vi "FindAccountView.vi"(1 "Exit Button":bool) -> (0 "error out":errorcluster caption="에러 출력")   [LabVIEW 2019]
uses:
  <vilib>/Utility/miscctls.llb/LVPointTypeDef.ctl
panel:
  in  "findType":enum32{"확인 버튼 2", "확인 버튼 3"}(radio)
  in  "findTab":enum32{"findIdTab", "findPwTab"}(tab)
  in  "idFindBtn":bool
  in  "idCancelBtn":bool
  in  "userNmForm":string caption="이름 *"
  in  "userEmailForm":string caption="이메일 *"
  in  "createdAtForm":string caption="가입일:"
  in  "문자열 3":string caption="아이디:"
  in  "userIdForm":string caption="아이디 *"
  in  "securityQuestion":string(combo) caption="보안 질문 선택 *"
  in  "securityAnswer":string caption="보안 질문 답변 *"
  in  "pwResetBtn":bool
  in  "pwCancelBtn":bool
  out "idChecK?":bool
  in  "정지":bool
  in  "error in (no error)":errorcluster caption="에러 입력(에러 없음)"
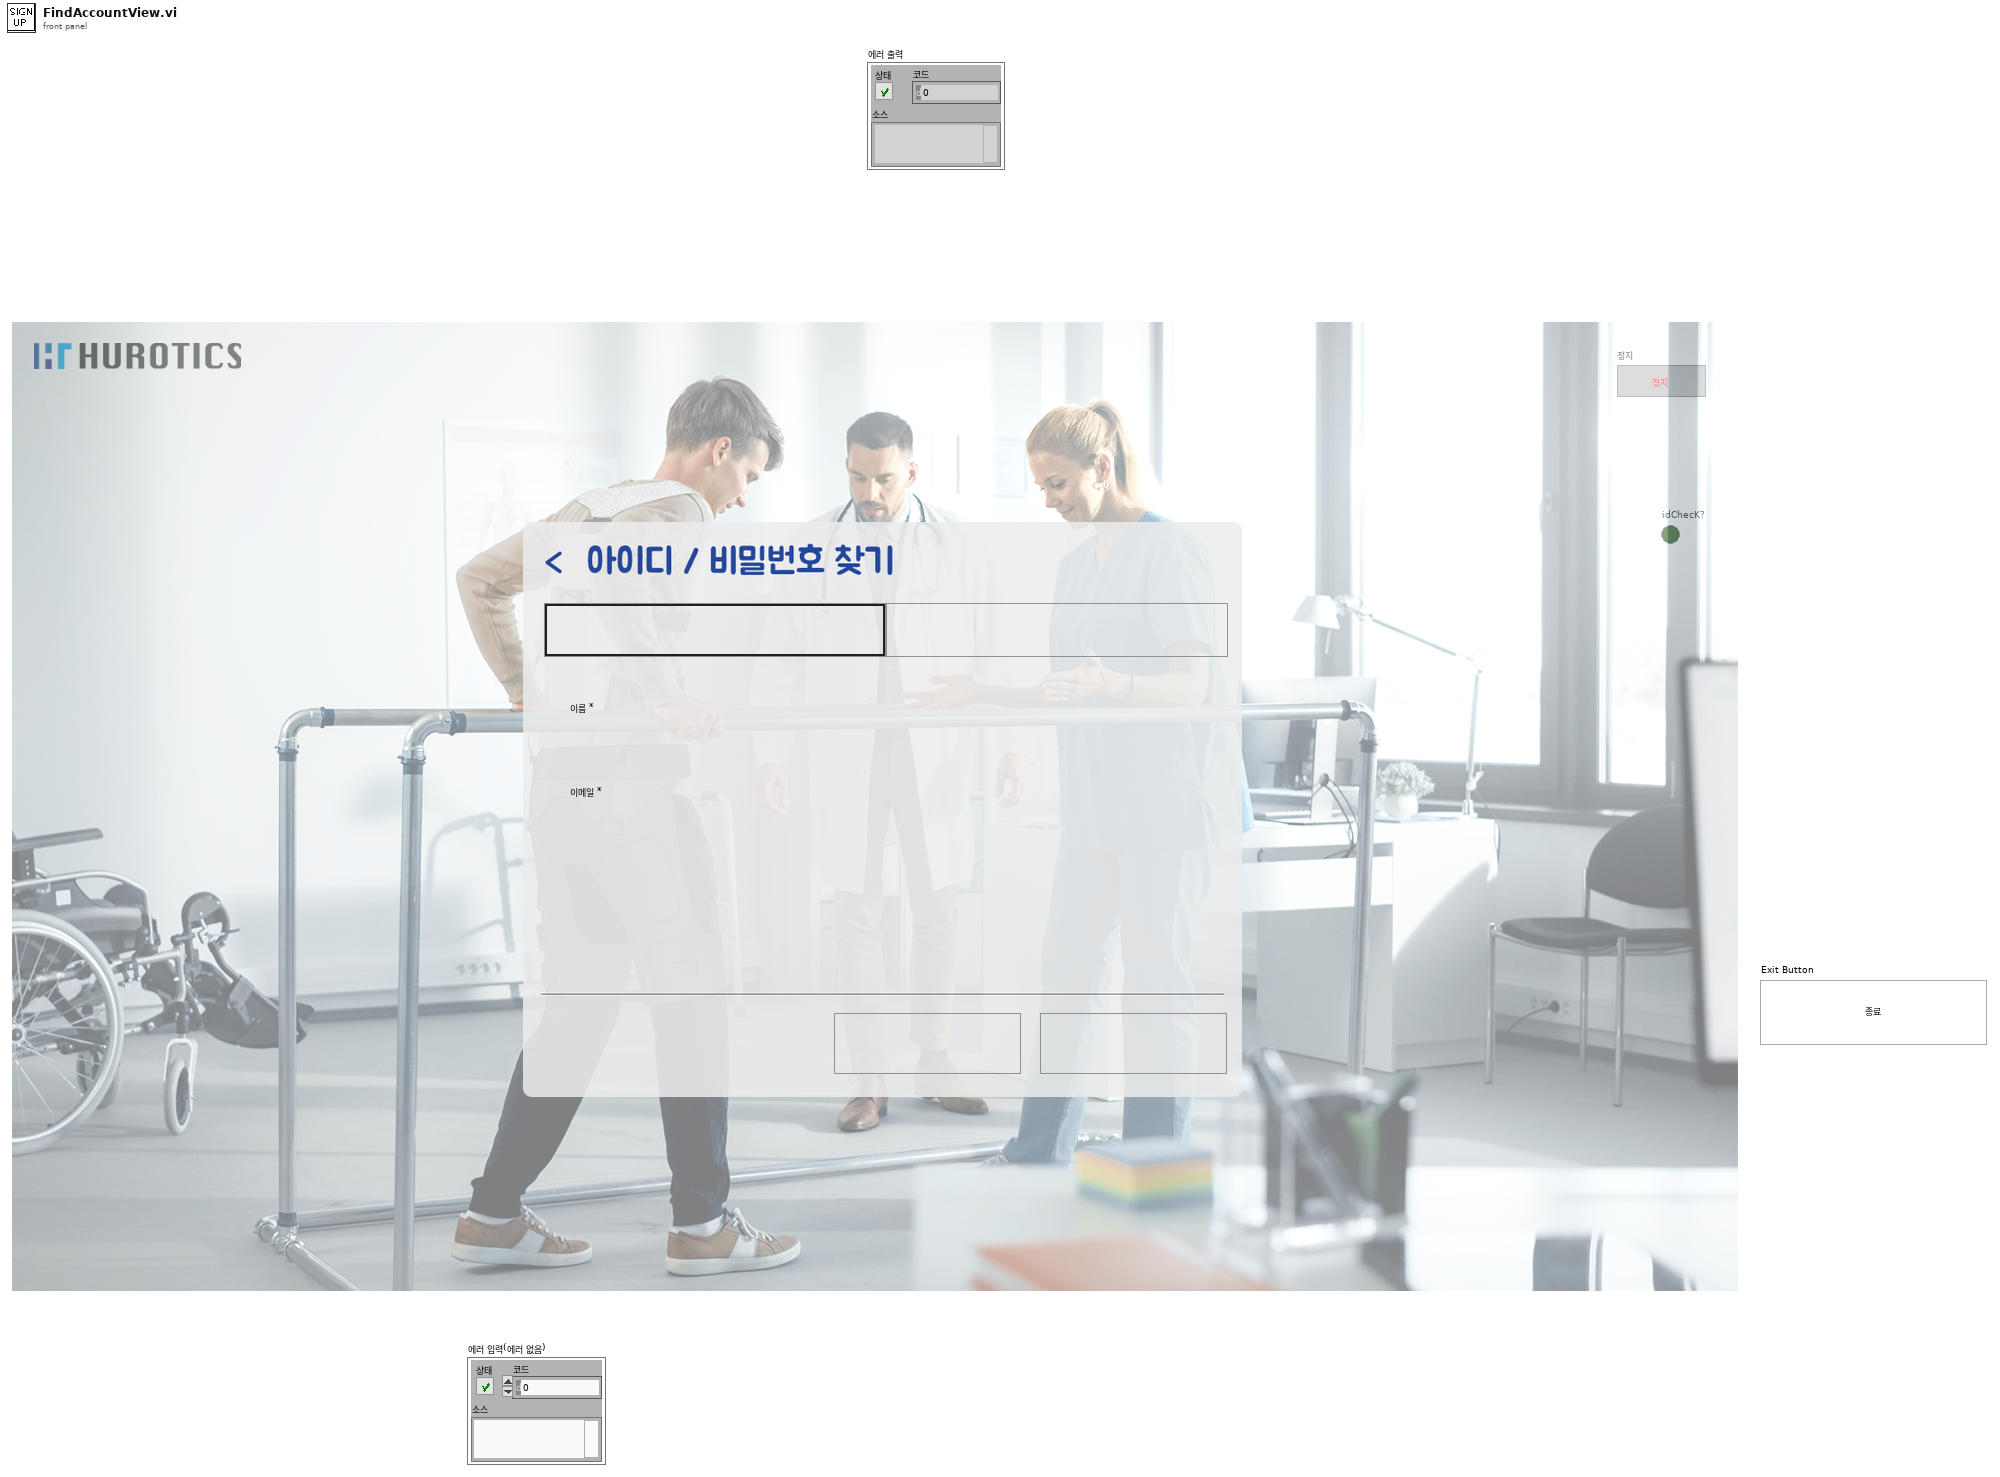
[diagram p1: front panel]
types:
  T1 = typedef "LVPointTypeDef.ctl" = cluster{"Horizontal":i16, "Vertical":i16}
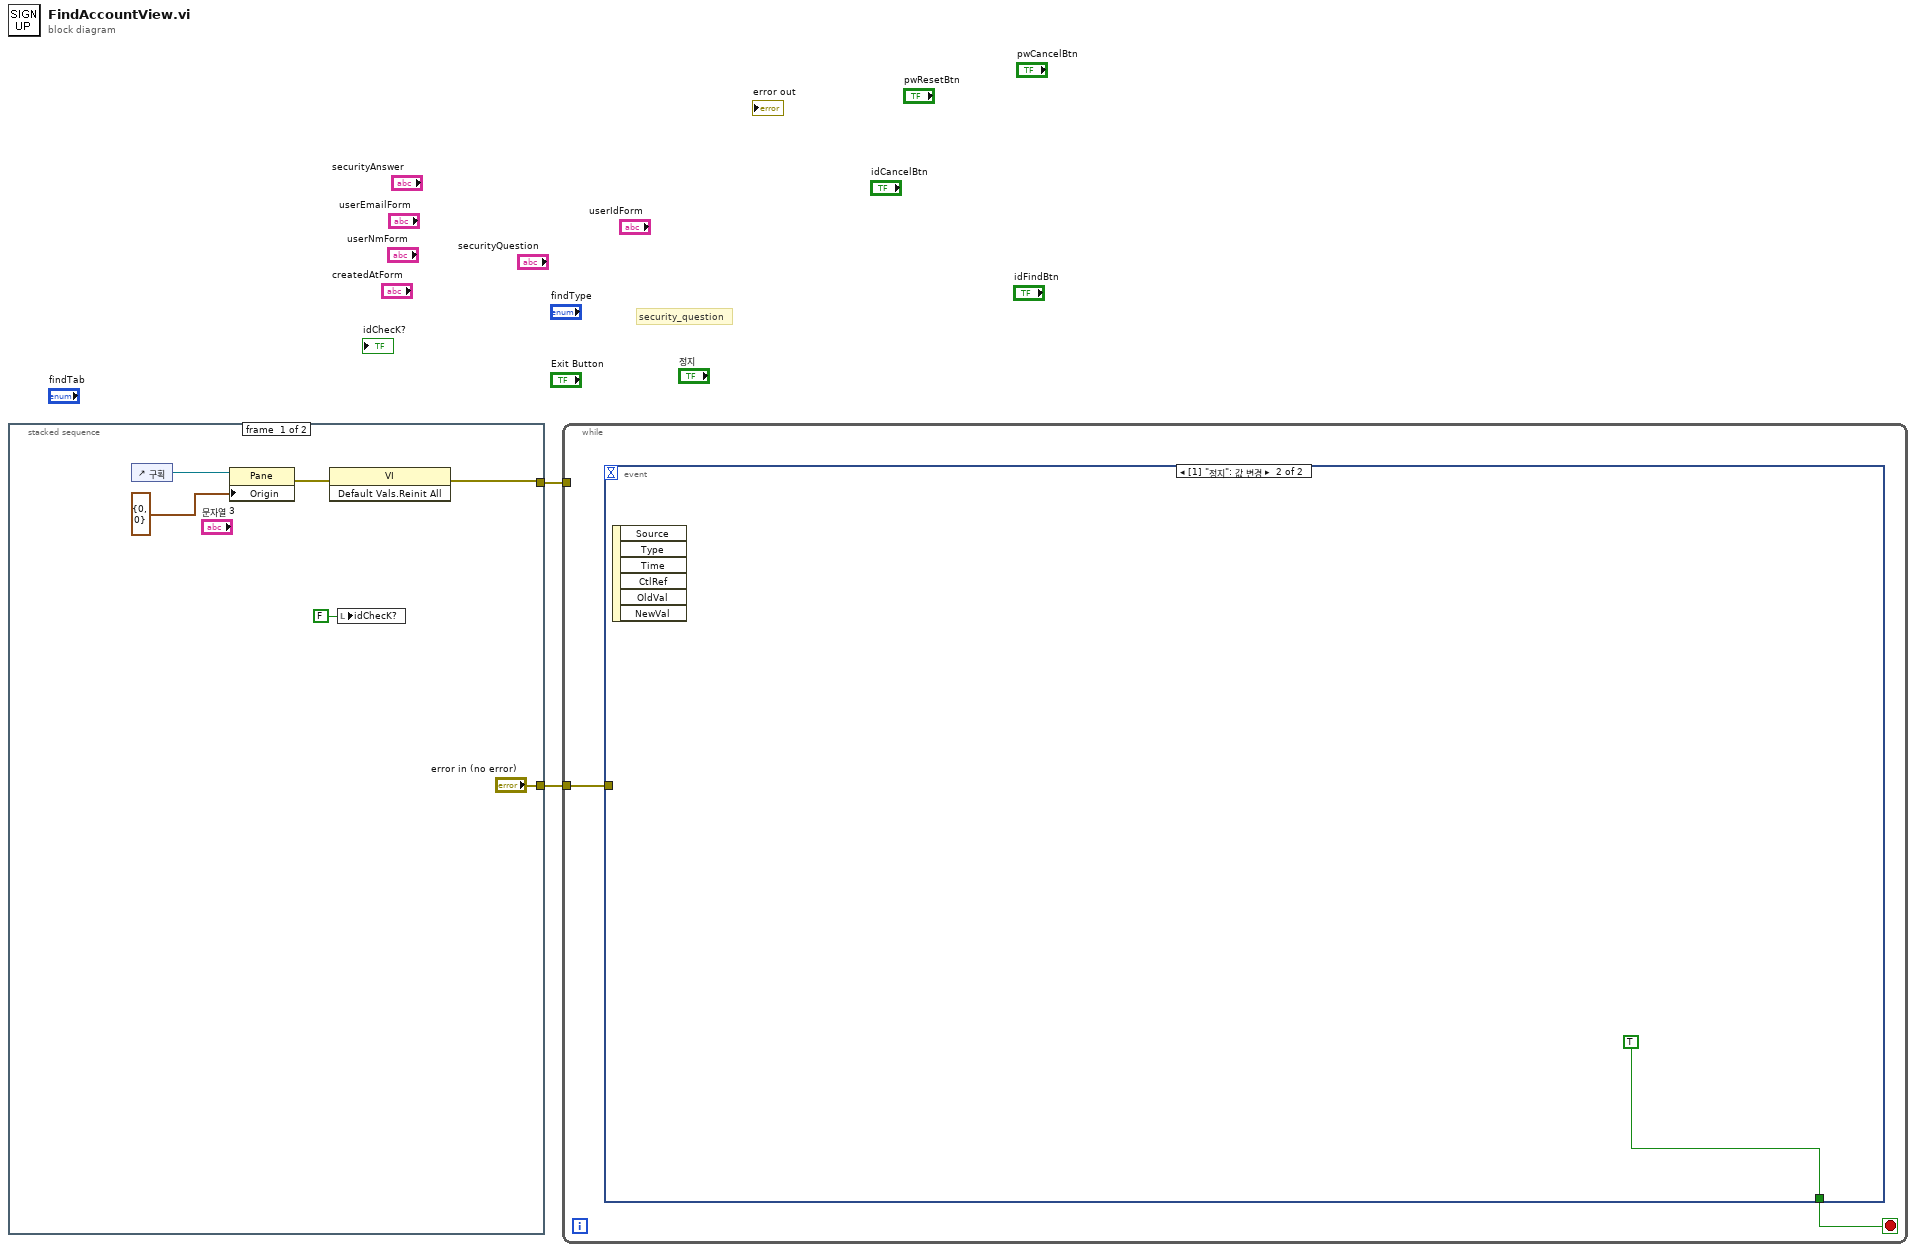
[diagram p0: block diagram]
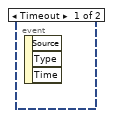
[diagram p3: hidden frame]
diagram:
  # "security_question"
  n1 = stacked-sequence {
    tunnel: ["error in (no error)" _] -> w2
    tunnel: [w4 _] -> w1
    frame #0 {
      n2 = control-ref of="구획"() -> (w7:refnum<vi>)
      n3 = property class="Pane"(reference=w7, "Origin"=T1 {"Horizontal"=0, "Vertical"=0} ("원점")) -> (error out=w6:errorcluster)  [unwired: 1 in, 1 out]
      n4 = invoke class="VI" method="Default Vals.Reinit All"(error in=w6) -> (error out=w4:errorcluster)  [unwired: 2 in, 2 out]
      n5 = local write "idChecK?"(FALSE ("idChecK?")) -> ()
    }
    frame #1 {
    }
  }
  n6 = while {
    tunnel: w2 -> [w9]
    tunnel: w1 -> [_]
    stop <- w10 stop-if-true
    n7 = event shown="[1] \"정지\": 값 변경" {
      selector: _ -> [_ _]
      dyn-events: _ -> [_ _]
      timeout: _ -> [_ _]
      tunnel: [_ TRUE] -> w10
      tunnel: w9 -> [_ _]
      event Timeout {
        n8 = event-data() -> ()  [unwired: 1 in, 3 out]
      }
      event "정지": Value Change {
        n9 = event-data() -> ()  [unwired: 1 in, 6 out]
      }
    }
  }
